vi "KM_file - read-write - list of lines.vi"(6 "append to file? (new file:F)":bool=TRUE, 7 "read/write control":T1=enum."append one line", 9 "header":string="frequency(Hz) Vx(V) Vy(V)", 10 "list of lines IN":string[](array[string])=["80565.153431138009\t0.000256949039\t-0.000315807330\t"], 11 "file path":path=path "C:/Data/December_2017/121317/9w/f004.dat") -> (1 "header OUT":string="frequency(Hz) Vx(V) Vy(V)", 2 "list of lines OUT":string[](array[string])=["80565.153431138009\t0.000256949039\t-0.000315807330\t"])   [LabVIEW 2018]
uses:
  file -- read-write control.ctl
  <vilib>/Utility/file.llb/Write Delimited Spreadsheet (string).vi
  <vilib>/Utility/file.llb/Read Delimited Spreadsheet (string).vi
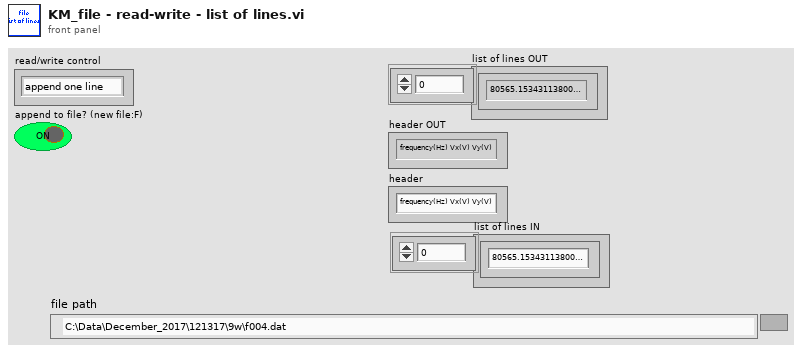
[diagram p1: front panel]
types:
  T1 = typedef "file -- read-write control.ctl" = enum16{"read", "write all", "append one line"}
  T2 = enum16{"open", "replace", "create", "open or create", "replace or create", "replace or create with confirmation"}
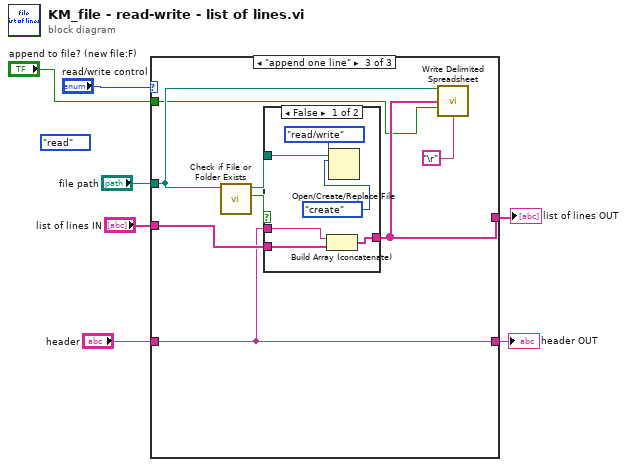
[diagram p0: block diagram]
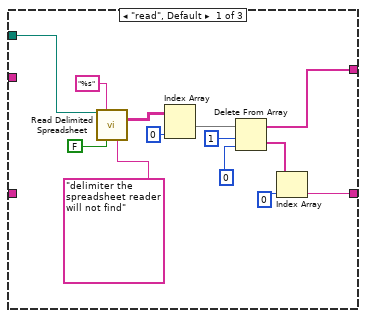
[diagram p2: hidden frame]
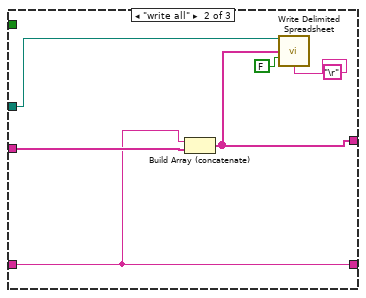
[diagram p3: hidden frame]
diagram:
  (unwired) file_--_read-write_control."read" ("read/write control")
  n1 = case shown="\"append one line\"" "read/write control" {
    tunnel: "file path" -> [w13 w24 w32]
    tunnel: [w9 w21 w28] -> w6
    tunnel: [w8 w22 w30] -> w5
    tunnel: "header" -> [_ w22 w30]
    tunnel: "list of lines IN" -> [_ w23 w31]
    tunnel: "append to file? (new file:F)" -> [_ _ w27]
    frame "read", Default {
      n2 = call-poly <vilib>:"Read Delimited Spreadsheet.vi"("file path (dialog if empty)"=w13, "format (%s)"="%s", "transpose? (F)"=FALSE ("append to file? (new file:F)"), "delimiter (\\t)"="delimiter the spreadsheet reader will not find" ("delimiter (\\t)")) -> ("all rows"=w18:string[][])  [unwired: 6 in, 5 out]
      n3 = Index Array(array=w18, index (col)=0 ("disabled index (col)")) -> (element=w16:string[])  [unwired: 1 in]
      n4 = Delete From Array(array=w16, length=1, index=0) -> (deleted portion=w11:string[], array with subset deleted=w9:string[])
      n5 = Index Array(array=w11, index=0 ("disabled index (col)")) -> (element=w8:string)
    }
    frame "write all" {
      n6 = Build Array (concatenate)(w22, w23) -> (w21:string[])
      n7 = call-poly <vilib>:"Write Delimited Spreadsheet.vi"("file path (dialog if empty)"=w24, "1D data"=w21, "append to file? (new file:F)"=FALSE, "delimiter (\\t)"="\r") -> ()  [unwired: 10 in, 2 out]
    }
    frame "append one line" {
      n8 = call <vilib>:"Check if File or Folder Exists.vi"("path"=w32) -> ("file or folder exists?"=w33:bool, "dup path"=w29:path)  [unwired: 8 in, 1 out]
      n9 = case shown="False" w33 {
        tunnel: w31 -> [w40 w41]
        tunnel: w30 -> [w39 _]
        tunnel: [w38 w41] -> w28
        tunnel: w29 -> [w37 _]
        frame False {
          n10 = Build Array (concatenate)(w39, w40) -> (w38:string[])
          n11 = Open/Create/Replace File(file path (use dialog)=w37, operation (0:open)=T2."create", access (0:read/write)=enum16{"read/write", "read-only", "write-only"}."read/write") -> ()  [unwired: 3 in, 3 out]
        }
        frame True {
        }
      }
      n12 = call-poly <vilib>:"Write Delimited Spreadsheet.vi"("file path (dialog if empty)"=w32, "1D data"=w28, "append to file? (new file:F)"=w27, "delimiter (\\t)"="\r") -> ()  [unwired: 10 in, 2 out]
    }
  }
  "list of lines OUT" <- w6
  "header OUT" <- w5
